vi "Turning_Power_Mode.vi"(8 "Turning_Scale":dbl=1.5 format="%#_13g", 9 "Quick_Turn":bool, 10 "Turning":dbl, 11 "Power":dbl) -> (3 "Turning_Correction":dbl)   [LabVIEW 2015]
panel:
  # "Turning_Power_Mode"
  # "This subsystem switches between speed based steering and normal steering"
  # "Tunning"
  # "Outputs"
  # "Inputs"
  # "Used to switch between steering modes"
  # "Adjust to compensate for  inertage a\n momentum allows for proper \nturning at high speeds"
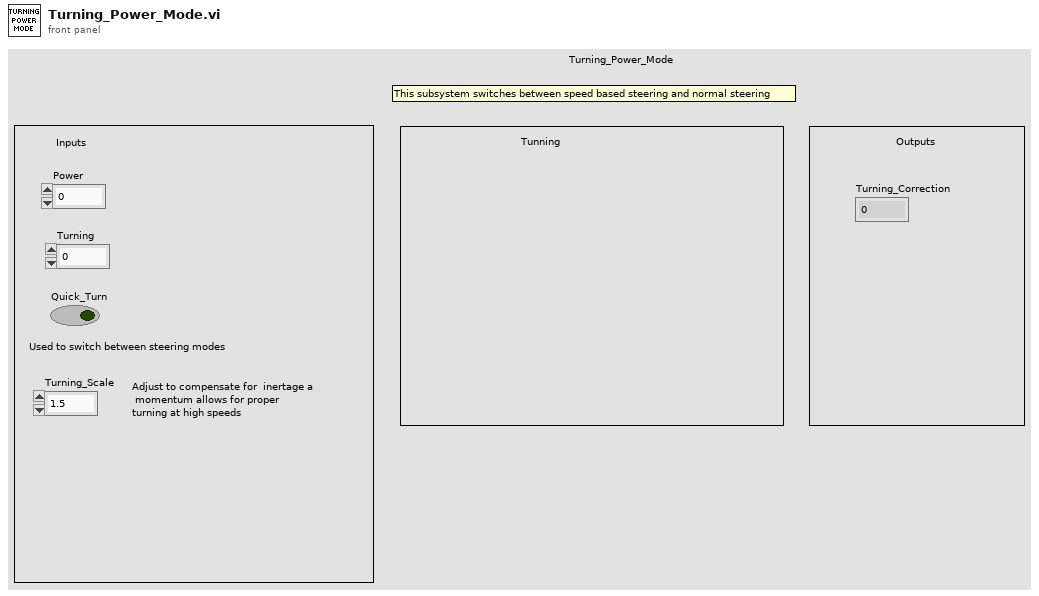
[diagram p1: front panel]
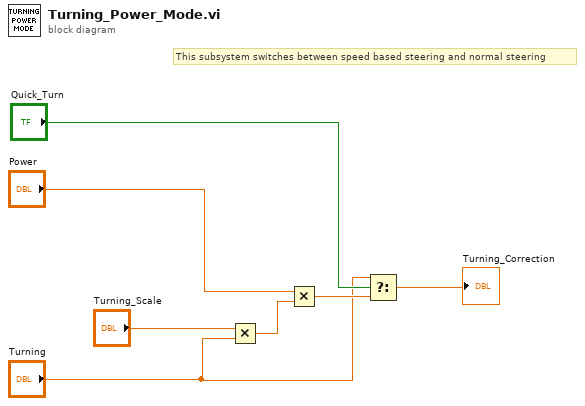
[diagram p0: block diagram]
diagram:
  # "This subsystem switches between speed based steering and normal steering"
  n1 = Multiply(x="Turning_Scale", y="Turning") -> (x*y=w7:dbl)
  n2 = Multiply(x="Power", y=w7) -> (x*y=w5:dbl)
  n3 = Select(t="Turning", s="Quick_Turn", f=w5) -> (s? t:f=→"Turning_Correction":dbl)
